vi "Read Server Port.vi"(8 "error in (no error)":errorcluster, 11 "Event_Syslog in":refnum<class "Event_Syslog.lvclass">) -> (0 "error out":errorcluster, 2 "Server Port":u16, 3 "Event_Syslog out":refnum<class "Event_Syslog.lvclass">)   [LabVIEW 2021, in "Event_Syslog.lvclass"]
uses:
  Event_Syslog.lvclass
  Event_Syslog.lvclass/Event_Syslog.ctl
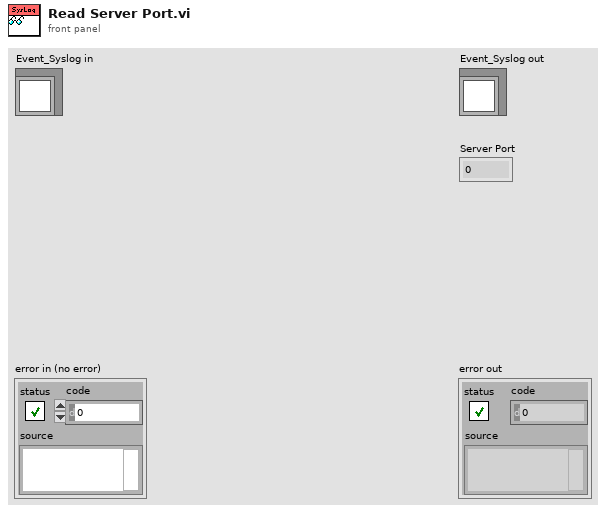
[diagram p1: front panel]
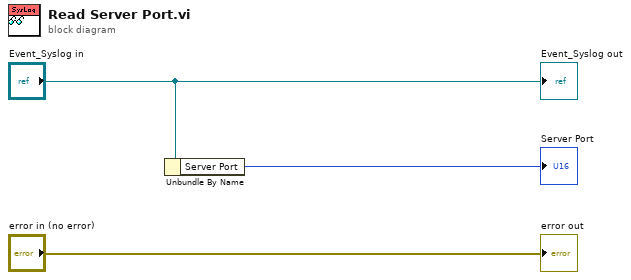
[diagram p0: block diagram]
diagram:
  n1 = Unbundle By Name("Event_Syslog in") -> ("Server Port"=→"Server Port":u16)
  "error out" <- "error in (no error)"
  "Event_Syslog out" <- "Event_Syslog in"
